vi "TimeLmtDialog_2Btn.vi"(9 "time(s)":i32=5, 10 "Infoin":string="在这里填写显示的信息内容", 11 "title":string="提示信息") -> (3 "OK?":bool)   [LabVIEW 2011]
panel:
  in  "cancel":bool
  in  "ok":bool
  out "info":string
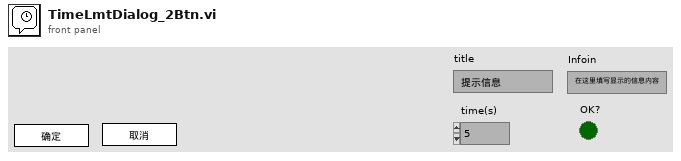
[diagram p1: front panel]
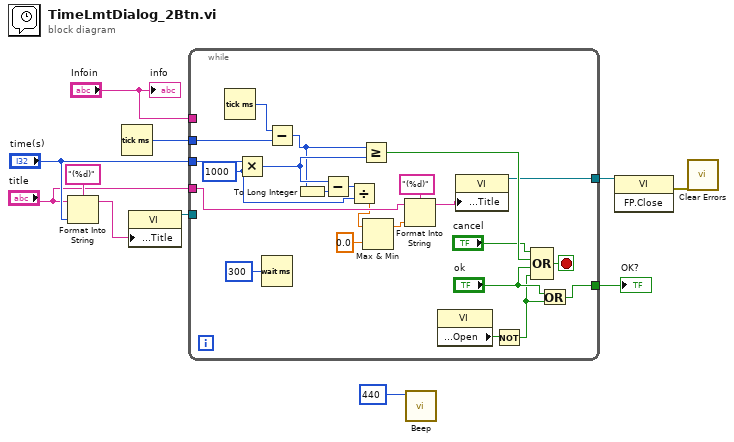
[diagram p0: block diagram]
diagram:
  n1 = Format Into String(format string="(%d)" ("格式字符串"), initial string="title", "time(s)") -> (resulting string=w7:string)  [unwired: 1 in, 1 out]
  n2 = Tick Count (ms)() -> (millisecond timer value=w5:u32)
  n3 = property class="VI"("Front Panel.Title"=w7) -> (reference out=w10:refnum<vi>)  [unwired: 2 in, 1 out]
  n4 = while {
    tunnel: "Infoin" -> [_]
    tunnel: "time(s)" -> [w31]
    tunnel: w10 -> [_]
    tunnel: "title" -> [w25]
    tunnel: w5 -> [w32]
    tunnel: [w18] -> w4
    tunnel: [w12] -> w1
    stop <- w15 stop-if-true
    w26 = 1000 ("y")
    n5 = Tick Count (ms)() -> (millisecond timer value=w33:u32)
    n6 = Multiply(x=w31, y=w26) -> (x*y=w29:i32)
    n7 = Wait (ms)(milliseconds to wait=u32 300 ("等待时间（毫秒）")) -> ()  [unwired: 1 out]
    n8 = Subtract(x=w33, y=w32) -> (x-y=w28:u32)
    n9 = To Long Integer(number=w28) -> (32bit integer=w19:i32)
    n10 = Subtract(x=w29, y=w19) -> (x-y=w27:i32)
    n11 = Divide(x=w27, y=w26) -> (x/y=w22:dbl)
    n12 = Greater Or Equal?(x=w28, y=w29) -> (x >= y?=w30:bool)
    n13 = Max & Min(x=w22, y=0.0) -> (max(x,y)=w20:dbl)  [unwired: 1 out]
    n14 = Format Into String(format string="(%d)" ("格式字符串"), initial string=w25, w20) -> (resulting string=w23:string)  [unwired: 1 in, 1 out]
    n15 = property class="VI"() -> ("Front Panel.Open"=w17:bool)  [unwired: 2 in, 2 out]
    n16 = property class="VI"("Front Panel.Title"=w23) -> (reference out=w18:refnum<vi>)  [unwired: 2 in, 1 out]
    n17 = Not(x=w17) -> (.not. x?=w13:bool)
    n18 = Compound Arithmetic op=OR("cancel", w30, "ok", w13) -> (w15:bool)
    n19 = Or(x="ok", y=w13) -> (x .or. y?=w12:bool)
  }
  "OK?" <- w1
  n20 = call <vilib>:"Beep.vi"("frequency (Hz)"=u32 440) -> ()  [unwired: 11 in]
  n21 = invoke class="VI" method="FP.Close"(reference=w4) -> (error out=w3:errorcluster)  [unwired: 2 in, 2 out]
  n22 = call <vilib>:"Clear Errors.vi"("error in (no error)"=w3) -> ()  [unwired: 6 in, 1 out]
  "info" <- "Infoin"
